vi "Yahoo - Raw Stock Data - Parse.vi"(0 "Raw Stock Data":string, 3 "error in":errorcluster) -> (7 "Stock Data":T1, 10 "error out":errorcluster)   [LabVIEW 2011]
doc: "Parse the Raw Stock Data to a cluster structure.\nThe expected Raw Stock Data format is:\n \"A\",\"Agilent Technolog\",42.68,+0.02,\"+0.05%\",2427956\n\nInputs:\n Raw Stock Data: Body of the HTTP request.\n Error in: Describes error conditions that occur before this node runs. This input provides standard error in functionality.\n\n\n\nOutputs:\n Stock Data: Parsed Stock Data\n Symbol\n Name\n Price\n Change\n Change %\n Volume: N/A\n Error out: Contains error information. This output provides standard error out functionality."
uses:
  Stock Data Control.ctl
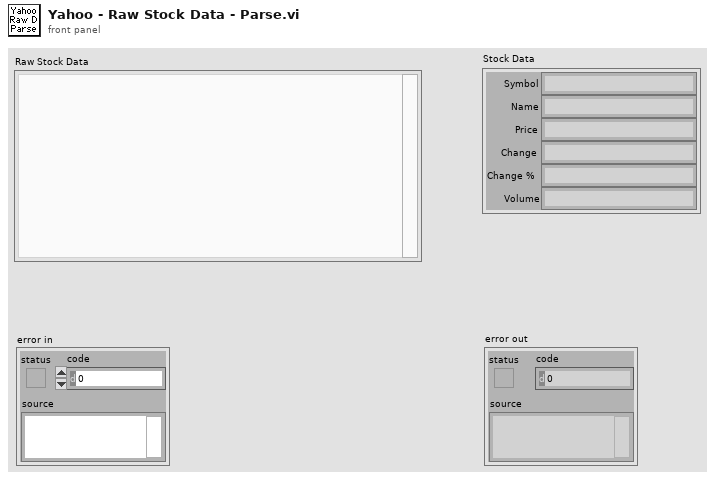
[diagram p1: front panel]
types:
  T1 = typedef "Stock Data Control.ctl" = cluster{"Symbol":string, "Name":string, "Price":string, "Change":string, "Change %":string, "Volume":string}
  T2 = cluster{"Symbol":string, "Name":string, "Price":string, "Change":string, "Change %":string, "Volume":string}
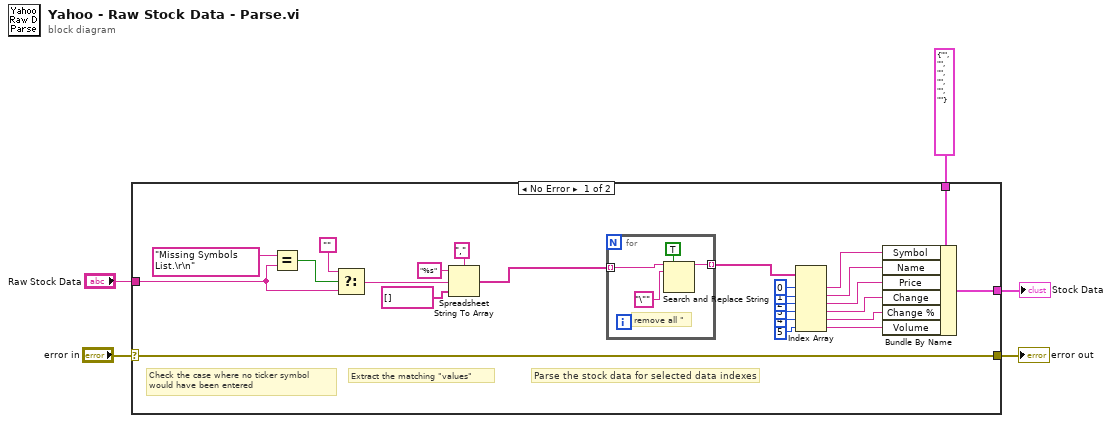
[diagram p0: block diagram]
diagram:
  n1 = case shown="No Error" "error in" {
    selector: "error in" -> [w30 w36]
    tunnel: [w30 w36] -> w4
    tunnel: "Raw Stock Data" -> [w7 _]
    tunnel: [w29 w35] -> w2
    tunnel: T2 {"Symbol"="", "Name"="", "Price"="", "Change"="", "Change %"="", "Volume"=""} ("Data") -> [w28 w35]
    frame No Error {
      # "Check the case where no ticker symbol\nwould have been entered"
      # "Extract the matching \"values\""
      # "Parse the stock data for selected data indexes"
      n2 = Equal?(x="Missing Symbols List.\r\n", y=w7) -> (x = y?=w8:bool)
      n3 = Select(t="", s=w8, f=w7) -> (s? t:f=w9:string)
      n4 = Spreadsheet String To Array(delimiter (Tab)=",", format string="%s", spreadsheet string=w9, array type (2D Dbl)=string[] []) -> (array=w11:string[])
      n5 = for {
        tunnel: [w33] -> w15 mode=indexing
        tunnel: w11 -> [w31] mode=indexing
        # "remove all \""
        n6 = Search and Replace String(replace all?=TRUE ("replace all? (F)"), input string=w31, search string="\"" ("format string")) -> (result string=w33:string)  [unwired: 5 in, 3 out]
      }
      n7 = Index Array(array=w15, index #1=0 ("index"), index #2=1 ("index"), index #3=2 ("index"), index #4=3 ("index"), index #5=4 ("index"), index #6=5 ("index")) -> (element #1=w23:string, element #2=w22:string, element #3=w21:string, element #4=w20:string, element #5=w17:string, element #6=w16:string)
      n8 = Bundle By Name(cluster=w28, "Symbol"=w23, "Name"=w22, "Price"=w21, "Change"=w20, "Change %"=w17, "Volume"=w16) -> (w29:T2)
    }
    frame Error {
    }
  }
  "error out" <- w4
  "Stock Data" <- w2
